vi "GDSLvIcon_GenerateObjectIcon.vi"(1 "HeaderColor":u32(colorbox)=786176, 3 "BackgroundColor":u32(colorbox)=16775072, 4 "Height":u32=22, 5 "error in (no error)":errorcluster, 6 "Type":enum16{"LvClass", "Library", "X-Control"}(ring), 7 "Width(30)":u32=30, 8 "ClassBodyIcon":string, 9 "_Thickness":u8=1 caption="Thickness (pixels)" min=1 max=3 step=1) -> (15 "BodyIconOut":u8[][](array[numeric])=[[2, 2, 2, 2, 2, 2, 2, 2, 2, 2, 2, 2, 2, 2, 2, 2, 2, 2, 2, 2, 2, 2, 2, 2, 2, 2, 2, 2, 2, 2], [2, 2, 2, 2, 2, 2, 2, 2, 2, 2, 2, 2, 2, 2, 185, 185, 2, 2, 2, 2, 2, 2, 2, 2, 2, 2, 2, 2, 2, 2], [2, 2, 2, 2, 2, 2, 2, 2, 2, 2, 2, 2, 185, 229, 227, 229, 229, 185, 2, 2, 2, 2, 2, 2, 2, 2, 2, 2, 2, 2], [2, 2, 2, 2, 2, 2, 2, 2, 2, 2, 185, 229, 227, 185, 185, 185, 185, 229, 229, 185, 2, 2, 2, 2, 2, 2, 2, 2, 2, 2], [2, 2, 2, 2, 2, 2, 2, 2, 185, 229, 227, 185, 185, 185, 185, 185, 185, 185, 185, 229, 229, 185, 2, 2, 2, 2, 2, 2, 2, 2], [2, 2, 2, 2, 2, 2, 2, 229, 227, 185, 185, 185, 185, 185, 185, 185, 185, 185, 185, 185, 185, 229, 229, 2, 2, 2, 2, 2, 2, 2], [2, 2, 2, 2, 2, 2, 2, 227, 227, 185, 185, 185, 185, 185, 185, 185, 185, 185, 185, 185, 185, 232, 229, 2, 2, 2, 2, 2, 2, 2], [2, 2, 2, 2, 2, 2, 2, 227, 229, 229, 227, 185, 185, 185, 185, 185, 185, 185, 185, 232, 232, 232, 227, 2, 2, 2, 2, 2, 2, 2], [2, 2, 2, 2, 2, 2, 2, 227, 229, 229, 229, 229, 227, 185, 185, 185, 185, 232, 232, 232, 232, 232, 227, 2, 2, 2, 2, 2, 2, 2], [2, 2, 2, 2, 2, 2, 2, 227, 229, 229, 229, 229, 229, 229, 227, 229, 232, 232, 232, 232, 232, 232, 227, 2, 2, 2, 2, 2, 2, 2], [2, 2, 2, 2, 2, 2, 2, 227, 229, 229, 229, 229, 229, 229, 229, 232, 232, 232, 232, 232, 232, 232, 227, 2, 2, 2, 2, 2, 2, 2], [2, 2, 2, 2, 2, 2, 2, 227, 229, 229, 229, 229, 229, 229, 229, 232, 232, 232, 232, 232, 232, 232, 227, 2, 2, 2, 2, 2, 2, 2], [2, 2, 2, 2, 2, 2, 2, 227, 229, 229, 229, 229, 229, 229, 229, 232, 232, 232, 232, 232, 232, 232, 227, 2, 2, 2, 2, 2, 2, 2], [2, 2, 2, 2, 2, 2, 2, 227, 229, 229, 229, 229, 229, 229, 229, 232, 232, 232, 232, 232, 232, 232, 227, 2, 2, 2, 2, 2, 2, 2], [2, 2, 2, 2, 2, 2, 2, 227, 229, 229, 229, 229, 229, 229, 229, 232, 232, 232, 232, 232, 232, 232, 227, 2, 2, 2, 2, 2, 2, 2], [2, 2, 2, 2, 2, 2, 2, 229, 229, 229, 229, 229, 229, 229, 229, 232, 232, 232, 232, 232, 232, 229, 229, 172, 172, 172, 2, 2, 2, 2], [2, 2, 2, 2, 2, 2, 2, 2, 227, 227, 229, 229, 229, 229, 229, 232, 232, 232, 232, 229, 229, 227, 172, 172, 172, 172, 172, 172, 2, 2], [2, 2, 2, 2, 2, 2, 2, 2, 2, 2, 227, 229, 229, 229, 229, 232, 232, 229, 229, 227, 172, 172, 172, 172, 172, 172, 2, 2, 2, 2], [2, 2, 2, 2, 2, 2, 2, 2, 2, 2, 2, 2, 227, 229, 229, 229, 229, 185, 172, 172, 172, 172, 172, 172, 172, 2, 2, 2, 2, 2], [2, 2, 2, 2, 2, 2, 2, 2, 2, 2, 2, 2, 2, 2, 227, 185, 172, 172, 172, 172, 172, 172, 172, 2, 2, 2, 2, 2, 2, 2], [2, 2, 2, 2, 2, 2, 2, 2, 2, 2, 2, 2, 2, 2, 2, 2, 2, 172, 172, 172, 172, 2, 2, 2, 2, 2, 2, 2, 2, 2], [2, 2, 2, 2, 2, 2, 2, 2, 2, 2, 2, 2, 2, 2, 2, 2, 2, 2, 2, 2, 2, 2, 2, 2, 2, 2, 2, 2, 2, 2]] format="%x", 19 "error out":errorcluster)   [LabVIEW 2020]
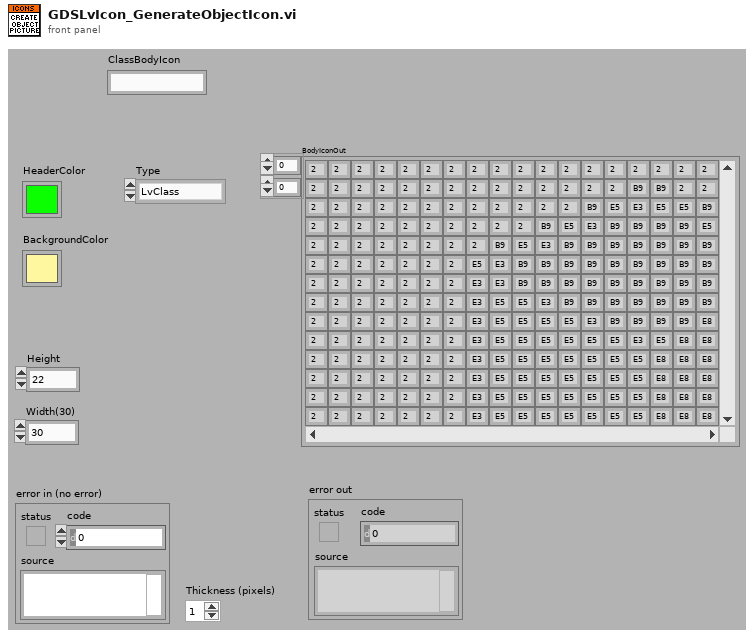
[diagram p1: front panel]
types:
  T1 = typedef "imagedata.ctl" = cluster{"image type":i32, "image depth":i32, "image":u8[], "mask":u8[], "colors":u32[], "Rectangle":cluster{"left":i16, "top":i16, "right":i16, "bottom":i16}}
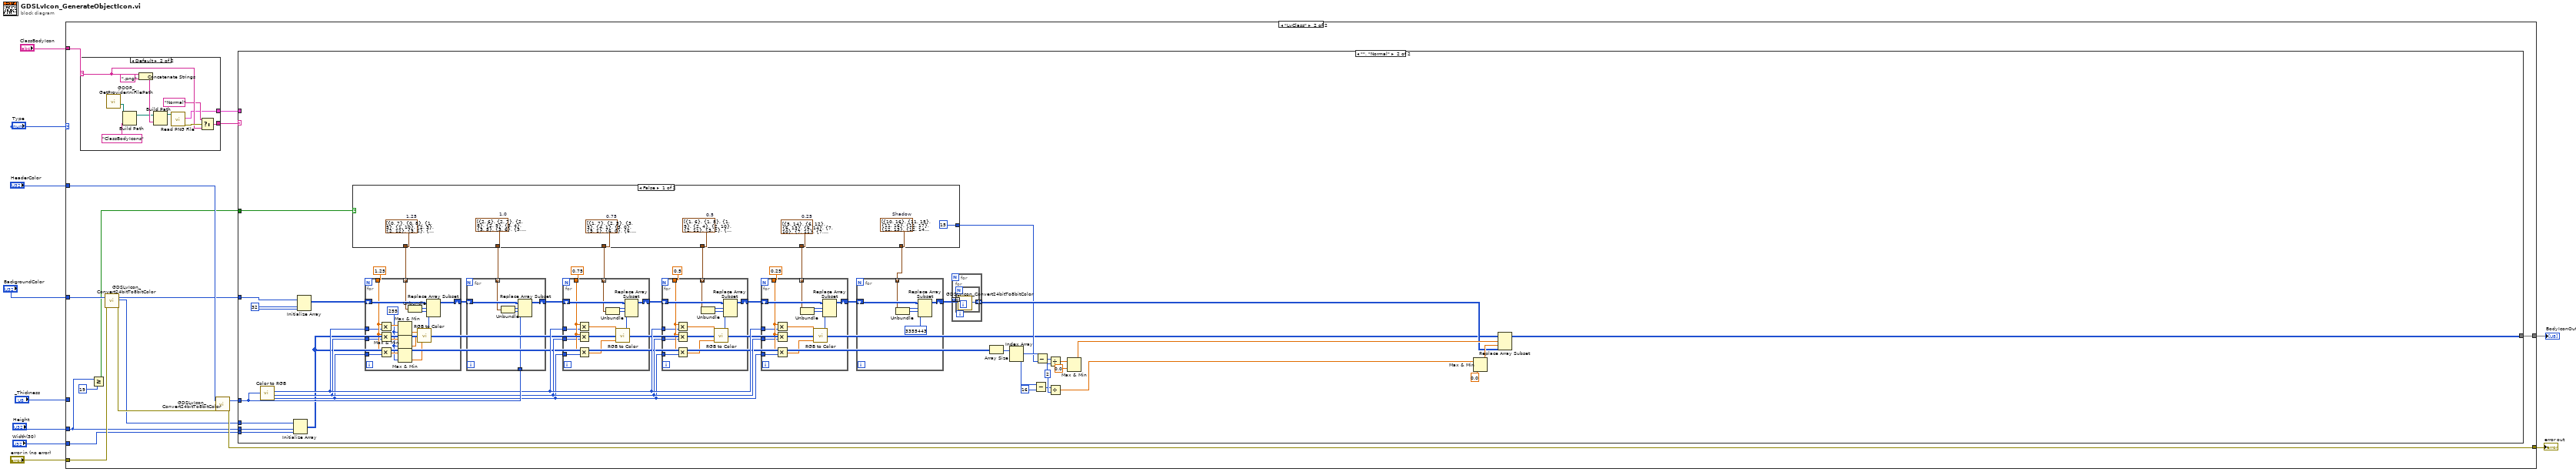
[diagram p0: block diagram]
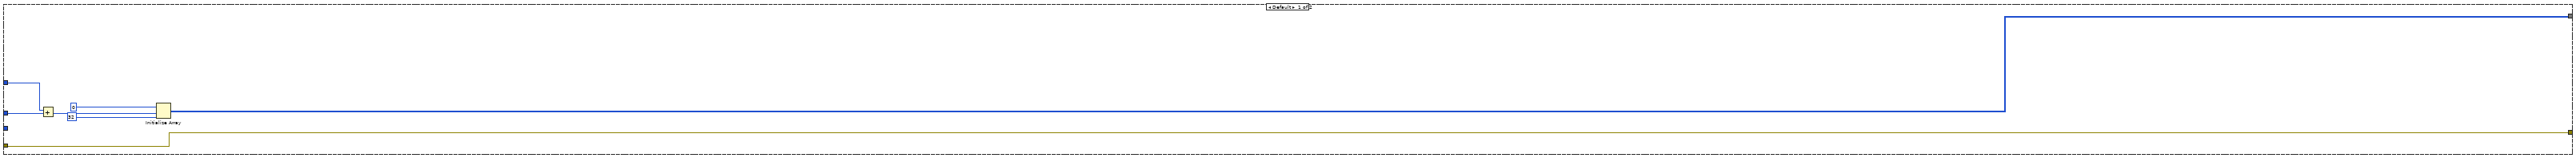
[diagram p2: hidden frame]
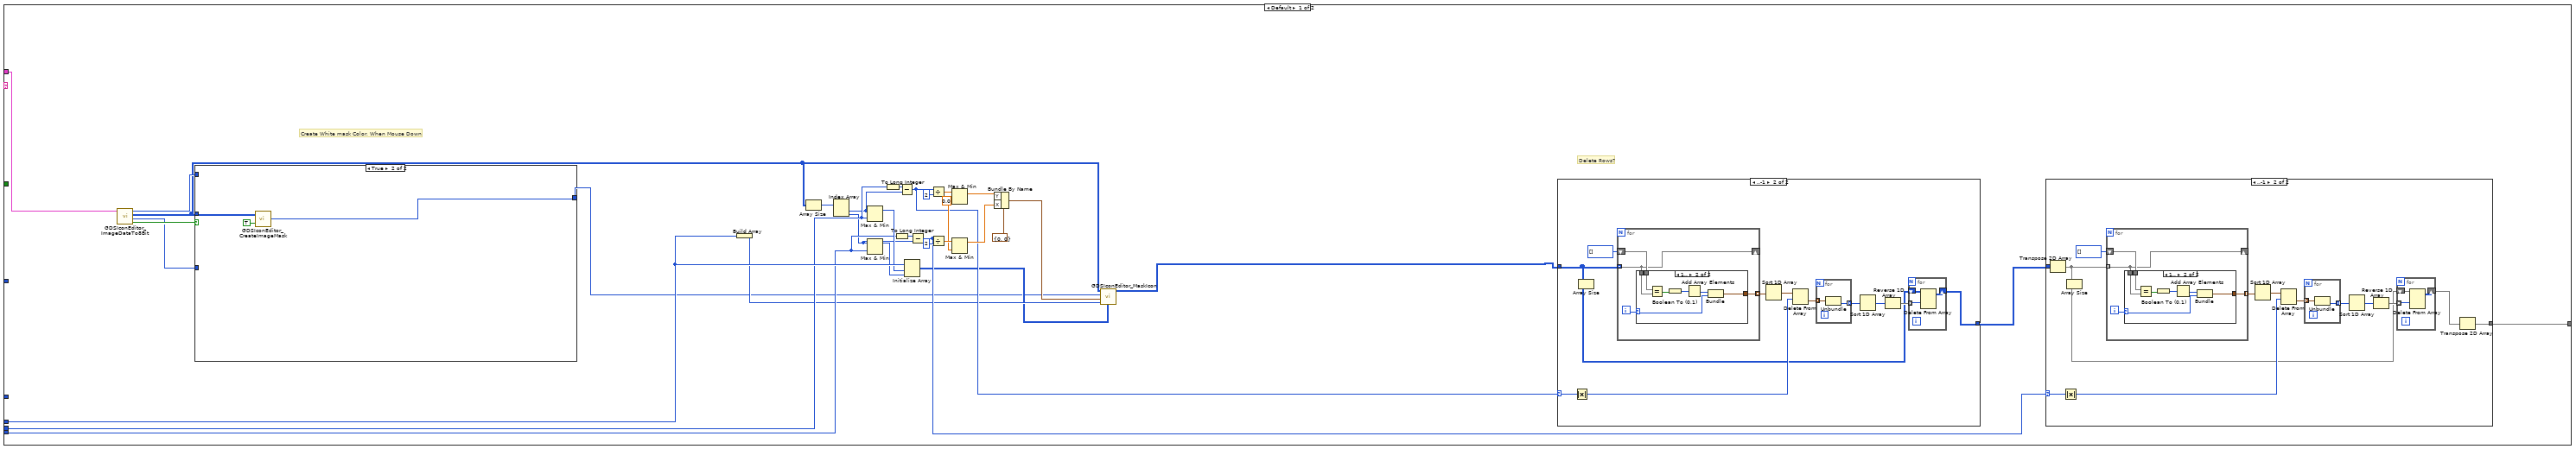
[diagram p4: hidden frame]
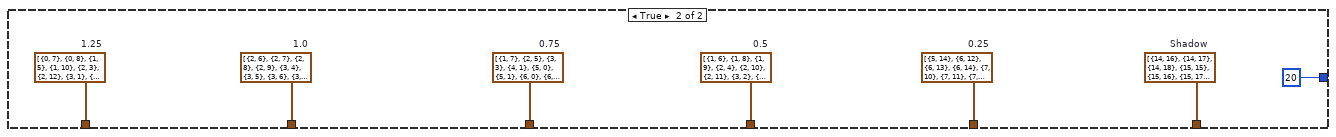
[diagram p10: hidden frame]
diagram:
  n1 = case shown="\"LvClass\"" "Type" {
    tunnel: "HeaderColor" -> [_ w33]
    tunnel: [w15 w31] -> w9
    tunnel: "BackgroundColor" -> [_ w30]
    tunnel: "error in (no error)" -> [w15 w29]
    tunnel: "Width(30)" -> [_ w18]
    tunnel: "Height" -> [w13 w19]
    tunnel: [w16 w22] -> w4
    tunnel: "_Thickness" -> [w12 _]
    tunnel: "ClassBodyIcon" -> [_ w24]
    frame Default {
      n2 = Add(x=w12, y=w13) -> (x+y=w11:u32)
      n3 = Initialize Array(u8 0 ("element"), w11, 32 ("dimension size")) -> (w16:u8[][])
    }
    frame "LvClass" {
      n4 = case shown="Default" w24 {
        selector: w24 -> [w34 w38]
        tunnel: [w34 w37] -> w23
        tunnel: [_ w35] -> w21
        frame "", "Normal" {
        }
        frame Default {
          n5 = call <resource>:"GOOP_GetProviderIniFilePath.vi"() -> ("ProviderMainFolder"=w42:path)  [unwired: 10 in, 1 out]
          n6 = Build Path(base path=w42, name or relative path="ClassBodyIcons") -> (appended path=w44:path)
          n7 = Concatenate Strings(w38, ".png" ("string")) -> (w45:string)
          n8 = Build Path(base path=w44, name or relative path=w45) -> (appended path=w40:path)
          n9 = call <vilib>:"Read PNG File.vi"("path to PNG file"=w40) -> ("error out"=w39:errorcluster, "image data"=w35:T1)  [unwired: 8 in, 1 out]
          n10 = Select(t="Normal", s=w39, f=w38) -> (s? t:f=w37:string)
        }
      }
      n11 = Greater Or Equal?(x=w19, y=19) -> (x >= y?=w26:bool)
      n12 = call <resource>:"GDSLvIcon_Convert24bitTo8bitColor.vi"("Color 24bit In"=w30, "error in (no error)"=w29) -> ("Adjusted 24bit Color Out"=w25:u32, "Color out(256)"=w20:u8, "error out"=w28:errorcluster)  [unwired: 14 in, 1 out]
      n13 = call <resource>:"GDSLvIcon_Convert24bitTo8bitColor.vi"("Color 24bit In"=w33, "error in (no error)"=w28) -> ("Adjusted 24bit Color Out"=w32:u32, "error out"=w31:errorcluster)  [unwired: 14 in, 2 out]
      n14 = case shown="\"\", \"Normal\"" w23 {
        tunnel: w32 -> [_ w180]
        tunnel: w26 -> [_ w162]
        tunnel: w25 -> [_ w161]
        tunnel: [w53 w144] -> w22
        tunnel: w21 -> [w75 _]
        tunnel: w20 -> [w73 w143]
        tunnel: w19 -> [w70 w142]
        tunnel: w18 -> [w62 w141]
        frame Default {
          w59 = 0.0 ("y")
          # "Delete Rows?"
          # "Create White mask Color, When Mouse Down"
          n15 = call <resource>:"GDSIconEditor_ImageDataTo8Bit.vi"("image data"=w75) -> ("NoMaskFound"=w77:bool, "ColorArray"=w52:u32[], "8-bit pixmap"=w49:u8[][], "mask"=w76:u8[])  [unwired: 7 in]
          n16 = case shown="True" w77 {
            tunnel: w49 -> [_ w139]
            tunnel: w76 -> [w136 _]
            tunnel: [w136 w137] -> w46
            tunnel: w52 -> [_ _]
            frame False {
            }
            frame True {
              n17 = call <resource>:"GDSIconEditor_CreateImageMask.vi"("Flood Fill"=TRUE, "8-bit pixmap"=w139) -> ("Array"=w137:u8[])
            }
          }
          n18 = Build Array(w73) -> (w50:u8[])
          n19 = Array Size(array=w49) -> (size(s)=w74:i32[])
          n20 = Index Array(array=w74) -> (element #1=w69:i32, element #2=w61:i32)  [unwired: 2 in]
          n21 = Max & Min(x=w69, y=w70) -> (max(x,y)=w72:u32)  [unwired: 1 out]
          n22 = Max & Min(x=w61, y=w62) -> (max(x,y)=w71:u32)  [unwired: 1 out]
          n23 = To Long Integer(number=w70) -> (32bit integer=w58:i32)
          n24 = To Long Integer(number=w62) -> (32bit integer=w57:i32)
          n25 = Subtract(x=w58, y=w69) -> (x-y=w56:i32)
          n26 = Initialize Array(w73, w72, w71) -> (w47:u8[][])
          n27 = Subtract(x=w57, y=w61) -> (x-y=w54:i32)
          n28 = Divide(x=w56, y=u32 2) -> (x/y=w67:dbl)
          n29 = Divide(x=w54, y=u32 2) -> (x/y=w64:dbl)
          n30 = Max & Min(x=w67, y=w59) -> (max(x,y)=w65:dbl)  [unwired: 1 out]
          n31 = Max & Min(x=w64, y=w59) -> (max(x,y)=w60:dbl)  [unwired: 1 out]
          n32 = Bundle By Name(cluster=cluster{"X":i32, "Y":i32} {"X"=0, "Y"=0} ("BgIconOffset"), "Y"=w65, "X"=w60) -> (w51:cluster{"X":i32, "Y":i32})
          n33 = call <resource>:"GDSIconEditor_MaskIcon.vi"("BgIcon"=w47, "ColorsOkayforiconToBeOnTopOf"=w50, "BgIconOffset"=w51, "BgIconMask"=w46, "IconIn"=w49) -> ("IconOut"=w48:u8[][])  [unwired: 6 in]
          n34 = case shown="..-1" w56 {
            selector: w56 -> [_ w119]
            tunnel: w48 -> [w108 w109]
            tunnel: [w108 w110] -> w55
            frame Default {
            }
            frame ..-1 {
              n35 = Absolute Value(x=w119) -> (abs(x)=w115:i32)
              n36 = Array Size(array=w109) -> ()  [unwired: 1 out]
              n37 = for {
                tunnel: w109 -> [w126] mode=indexing
                shift-right: [w126] -> _
                shift-left: u8[] [] -> [w127]
                tunnel: [w125] -> w117 mode=indexing
                i -> [w128]
                n38 = case shown="1.." w128 {
                  selector: w128 -> [_ w130]
                  tunnel: w127 -> [_ w135]
                  tunnel: w126 -> [_ w134]
                  tunnel: [_ w129] -> w125
                  frame 0, Default {
                  }
                  frame 1.. {
                    n39 = Equal?(x=w135, y=w134) -> (x = y?=w133:bool[])
                    n40 = Boolean To (0,1)(Boolean=w133) -> (0, 1=w132:i16[])
                    n41 = Add Array Elements(numeric array=w132) -> (sum=w131:i16)
                    n42 = Bundle("Color out(256)"=w131, w130) -> (w129:cluster{"Color out(256)":i16, i32})  [unwired: 1 in]
                  }
                }
              }
              n43 = Sort 1D Array(array=w117) -> (sorted array=w116:cluster{"Color out(256)":i16, i32}[])
              n44 = Delete From Array(array=w116, length=w115) -> (deleted portion=w114:cluster{"Color out(256)":i16, i32}[])  [unwired: 1 in, 1 out]
              n45 = for {
                tunnel: w114 -> [w124] mode=indexing
                tunnel: [w123] -> w113 mode=indexing
                n46 = Unbundle(w124) -> (w123:i32)  [unwired: 1 out]
              }
              n47 = Sort 1D Array(array=w113) -> (sorted array=w112:i32[])
              n48 = Reverse 1D Array(array=w112) -> (reversed array=w111:i32[])
              n49 = for {
                tunnel: w111 -> [w120] mode=indexing
                shift-right: [w121] -> w110
                shift-left: w109 -> [w122]
                n50 = Delete From Array(array=w122, index (row)=w120) -> (array with subset deleted=w121:u8[][])  [unwired: 2 in, 1 out]
              }
            }
          }
          n51 = case shown="..-1" w54 {
            selector: w54 -> [_ w91]
            tunnel: w55 -> [w78 w81]
            tunnel: [w78 w79] -> w53
            frame Default {
            }
            frame ..-1 {
              n52 = Transpose 2D Array(2D array=w81) -> (transposed array=w80:u8[][])
              n53 = Absolute Value(x=w91) -> (abs(x)=w87:i32)
              n54 = Array Size(array=w80) -> ()  [unwired: 1 out]
              n55 = for {
                tunnel: w80 -> [w98] mode=indexing
                shift-right: [w98] -> _
                shift-left: u8[] [] -> [w99]
                tunnel: [w97] -> w89 mode=indexing
                i -> [w100]
                n56 = case shown="1.." w100 {
                  selector: w100 -> [_ w102]
                  tunnel: w99 -> [_ w107]
                  tunnel: w98 -> [_ w106]
                  tunnel: [_ w101] -> w97
                  frame 0, Default {
                  }
                  frame 1.. {
                    n57 = Equal?(x=w107, y=w106) -> (x = y?=w105:bool[])
                    n58 = Boolean To (0,1)(Boolean=w105) -> (0, 1=w104:i16[])
                    n59 = Add Array Elements(numeric array=w104) -> (sum=w103:i16)
                    n60 = Bundle("Color out(256)"=w103, w102) -> (w101:cluster{"Color out(256)":i16, i32})  [unwired: 1 in]
                  }
                }
              }
              n61 = Sort 1D Array(array=w89) -> (sorted array=w88:cluster{"Color out(256)":i16, i32}[])
              n62 = Delete From Array(array=w88, length=w87) -> (deleted portion=w86:cluster{"Color out(256)":i16, i32}[])  [unwired: 1 in, 1 out]
              n63 = for {
                tunnel: w86 -> [w96] mode=indexing
                tunnel: [w95] -> w85 mode=indexing
                n64 = Unbundle(w96) -> (w95:i32)  [unwired: 1 out]
              }
              n65 = Sort 1D Array(array=w85) -> (sorted array=w84:i32[])
              n66 = Reverse 1D Array(array=w84) -> (reversed array=w83:i32[])
              n67 = for {
                tunnel: w83 -> [w92] mode=indexing
                shift-right: [w93] -> w82
                shift-left: w80 -> [w94]
                n68 = Delete From Array(array=w94, index (row)=w92) -> (array with subset deleted=w93:u8[][])  [unwired: 2 in, 1 out]
              }
              n69 = Transpose 2D Array(2D array=w82) -> (transposed array=w79:u8[][])
            }
          }
        }
        frame "", "Normal" {
          w151 = 2 ("y")
          w169 = 32 ("dimension size")
          n70 = call <vilib>:"Color to RGB.vi"("Color"=w180) -> ("R"=w172:u8, "G"=w171:u8, "B"=w170:u8)  [unwired: 1 out]
          n71 = Initialize Array(w143, w142, w141) -> (w140:u8[][])
          n72 = Initialize Array(w161, w169, w169) -> (w183:u32[][])
          n73 = case shown="False" w162 {
            tunnel: [w189 w201] -> w168
            tunnel: [w190 w200] -> w167
            tunnel: [w191 w199] -> w166
            tunnel: [w192 w198] -> w165
            tunnel: [w193 w197] -> w164
            tunnel: [w194 w196] -> w163
            tunnel: [15 ("y") 20 ("y")] -> w145
            frame False {
              w189 = cluster{"X":i32, "Y":i32}[] [{"X"=0, "Y"=7}, {"X"=0, "Y"=8}, {"X"=1, "Y"=5}, {"X"=1, "Y"=10}, {"X"=2, "Y"=3}, {"X"=2, "Y"=12}, {"X"=3, "Y"=1}, {"X"=3, "Y"=14}]  # 1.25
              w190 = cluster{"X":i32, "Y":i32}[] [{"X"=2, "Y"=6}, {"X"=2, "Y"=7}, {"X"=2, "Y"=8}, {"X"=2, "Y"=9}, {"X"=3, "Y"=4}, {"X"=3, "Y"=5}, {"X"=3, "Y"=6}, {"X"=3, "Y"=7}, {"X"=3, "Y"=8}, {"X"=3, "Y"=9}, {"X"=3, "Y"=10}, {"X"=3, "Y"=11}, {"X"=4, "Y"=2}, {"X"=4, "Y"=3}, {"X"=4, "Y"=4}, {"X"=4, "Y"=5}, {"X"=4, "Y"=6}, {"X"=4, "Y"=7}, {"X"=4, "Y"=8}, {"X"=4, "Y"=9}, {"X"=4, "Y"=10}, {"X"=4, "Y"=11}, {"X"=4, "Y"=12}, {"X"=4, "Y"=13}, {"X"=5, "Y"=2}, {"X"=5, "Y"=3}, {"X"=5, "Y"=4}, {"X"=5, "Y"=5}, {"X"=5, "Y"=6}, {"X"=5, "Y"=7}, {"X"=5, "Y"=8}, {"X"=5, "Y"=9}, {"X"=5, "Y"=10}, {"X"=5, "Y"=11}, {"X"=5, "Y"=12}, {"X"=5, "Y"=13}, {"X"=6, "Y"=4}, {"X"=6, "Y"=5}, {"X"=6, "Y"=6}, {"X"=6, "Y"=7}, {"X"=6, "Y"=8}, {"X"=6, "Y"=9}, {"X"=6, "Y"=10}, {"X"=6, "Y"=11}, {"X"=7, "Y"=6}, {"X"=7, "Y"=7}, {"X"=7, "Y"=8}, {"X"=7, "Y"=9}, {"X"=13, "Y"=10}, {"X"=14, "Y"=8}]  # 1.0
              w192 = cluster{"X":i32, "Y":i32}[] [{"X"=1, "Y"=6}, {"X"=1, "Y"=8}, {"X"=1, "Y"=9}, {"X"=2, "Y"=4}, {"X"=2, "Y"=10}, {"X"=2, "Y"=11}, {"X"=3, "Y"=2}, {"X"=3, "Y"=12}, {"X"=3, "Y"=13}, {"X"=4, "Y"=0}, {"X"=4, "Y"=14}, {"X"=4, "Y"=15}, {"X"=5, "Y"=15}, {"X"=6, "Y"=1}, {"X"=6, "Y"=2}, {"X"=7, "Y"=1}, {"X"=7, "Y"=2}, {"X"=7, "Y"=3}, {"X"=7, "Y"=4}, {"X"=8, "Y"=1}, {"X"=8, "Y"=2}, {"X"=8, "Y"=3}, {"X"=8, "Y"=4}, {"X"=8, "Y"=5}, {"X"=8, "Y"=6}, {"X"=8, "Y"=8}, {"X"=9, "Y"=1}, {"X"=9, "Y"=2}, {"X"=9, "Y"=3}, {"X"=9, "Y"=4}, {"X"=9, "Y"=5}, {"X"=9, "Y"=6}, {"X"=9, "Y"=7}, {"X"=10, "Y"=0}, {"X"=10, "Y"=1}, {"X"=10, "Y"=2}, {"X"=10, "Y"=3}, {"X"=10, "Y"=4}, {"X"=10, "Y"=5}, {"X"=10, "Y"=6}, {"X"=10, "Y"=7}, {"X"=10, "Y"=14}, {"X"=10, "Y"=15}, {"X"=11, "Y"=3}, {"X"=11, "Y"=4}, {"X"=11, "Y"=5}, {"X"=11, "Y"=6}, {"X"=11, "Y"=7}, {"X"=11, "Y"=12}, {"X"=11, "Y"=13}, {"X"=12, "Y"=4}, {"X"=12, "Y"=5}, {"X"=12, "Y"=6}, {"X"=12, "Y"=7}, {"X"=12, "Y"=10}, {"X"=12, "Y"=11}, {"X"=13, "Y"=6}, {"X"=13, "Y"=7}, {"X"=13, "Y"=8}, {"X"=13, "Y"=9}]  # 0.5
              w191 = cluster{"X":i32, "Y":i32}[] [{"X"=1, "Y"=7}, {"X"=2, "Y"=5}, {"X"=3, "Y"=3}, {"X"=4, "Y"=1}, {"X"=5, "Y"=0}, {"X"=5, "Y"=1}, {"X"=6, "Y"=0}, {"X"=6, "Y"=3}, {"X"=6, "Y"=15}, {"X"=7, "Y"=0}, {"X"=7, "Y"=5}, {"X"=7, "Y"=15}, {"X"=8, "Y"=0}, {"X"=8, "Y"=7}, {"X"=8, "Y"=15}, {"X"=9, "Y"=0}, {"X"=9, "Y"=15}, {"X"=11, "Y"=1}, {"X"=11, "Y"=2}, {"X"=11, "Y"=14}, {"X"=12, "Y"=3}, {"X"=12, "Y"=12}, {"X"=13, "Y"=5}, {"X"=14, "Y"=7}]  # 0.75
              w193 = cluster{"X":i32, "Y":i32}[] [{"X"=5, "Y"=14}, {"X"=6, "Y"=12}, {"X"=6, "Y"=13}, {"X"=6, "Y"=14}, {"X"=7, "Y"=10}, {"X"=7, "Y"=11}, {"X"=7, "Y"=12}, {"X"=7, "Y"=13}, {"X"=7, "Y"=14}, {"X"=8, "Y"=9}, {"X"=8, "Y"=10}, {"X"=8, "Y"=11}, {"X"=8, "Y"=12}, {"X"=8, "Y"=13}, {"X"=8, "Y"=14}, {"X"=9, "Y"=8}, {"X"=9, "Y"=9}, {"X"=9, "Y"=10}, {"X"=9, "Y"=11}, {"X"=9, "Y"=12}, {"X"=9, "Y"=13}, {"X"=9, "Y"=14}, {"X"=10, "Y"=8}, {"X"=10, "Y"=9}, {"X"=10, "Y"=10}, {"X"=10, "Y"=11}, {"X"=10, "Y"=12}, {"X"=10, "Y"=13}, {"X"=11, "Y"=8}, {"X"=11, "Y"=9}, {"X"=11, "Y"=10}, {"X"=11, "Y"=11}, {"X"=12, "Y"=8}, {"X"=12, "Y"=9}]  # 0.25
              w194 = cluster{"X":i32, "Y":i32}[] [{"X"=10, "Y"=16}, {"X"=11, "Y"=15}, {"X"=11, "Y"=16}, {"X"=11, "Y"=17}, {"X"=12, "Y"=13}, {"X"=12, "Y"=14}, {"X"=12, "Y"=15}, {"X"=12, "Y"=16}, {"X"=12, "Y"=17}, {"X"=13, "Y"=11}, {"X"=13, "Y"=12}, {"X"=13, "Y"=13}, {"X"=13, "Y"=14}, {"X"=13, "Y"=15}, {"X"=13, "Y"=16}, {"X"=14, "Y"=9}, {"X"=14, "Y"=10}, {"X"=14, "Y"=11}, {"X"=14, "Y"=12}, {"X"=14, "Y"=13}, {"X"=14, "Y"=14}, {"X"=14, "Y"=15}, {"X"=15, "Y"=10}, {"X"=15, "Y"=11}, {"X"=15, "Y"=12}, {"X"=15, "Y"=13}]  # Shadow
            }
            frame True {
              w196 = cluster{"X":i32, "Y":i32}[] [{"X"=14, "Y"=16}, {"X"=14, "Y"=17}, {"X"=14, "Y"=18}, {"X"=15, "Y"=15}, {"X"=15, "Y"=16}, {"X"=15, "Y"=17}, {"X"=15, "Y"=18}, {"X"=15, "Y"=19}, {"X"=15, "Y"=20}, {"X"=16, "Y"=13}, {"X"=16, "Y"=14}, {"X"=16, "Y"=15}, {"X"=16, "Y"=16}, {"X"=16, "Y"=17}, {"X"=16, "Y"=18}, {"X"=17, "Y"=11}, {"X"=17, "Y"=12}, {"X"=17, "Y"=13}, {"X"=17, "Y"=14}, {"X"=17, "Y"=15}, {"X"=17, "Y"=16}, {"X"=17, "Y"=17}, {"X"=18, "Y"=9}, {"X"=18, "Y"=10}, {"X"=18, "Y"=11}, {"X"=18, "Y"=12}, {"X"=18, "Y"=13}, {"X"=18, "Y"=14}, {"X"=18, "Y"=15}, {"X"=19, "Y"=10}, {"X"=19, "Y"=11}, {"X"=19, "Y"=12}, {"X"=19, "Y"=13}]  # Shadow
              w197 = cluster{"X":i32, "Y":i32}[] [{"X"=5, "Y"=14}, {"X"=6, "Y"=12}, {"X"=6, "Y"=13}, {"X"=6, "Y"=14}, {"X"=7, "Y"=10}, {"X"=7, "Y"=11}, {"X"=7, "Y"=12}, {"X"=7, "Y"=13}, {"X"=7, "Y"=14}, {"X"=8, "Y"=9}, {"X"=8, "Y"=10}, {"X"=8, "Y"=11}, {"X"=8, "Y"=12}, {"X"=8, "Y"=13}, {"X"=8, "Y"=14}, {"X"=9, "Y"=8}, {"X"=9, "Y"=9}, {"X"=9, "Y"=10}, {"X"=9, "Y"=11}, {"X"=9, "Y"=12}, {"X"=9, "Y"=13}, {"X"=9, "Y"=14}, {"X"=10, "Y"=8}, {"X"=10, "Y"=9}, {"X"=10, "Y"=10}, {"X"=10, "Y"=11}, {"X"=10, "Y"=12}, {"X"=10, "Y"=13}, {"X"=10, "Y"=14}, {"X"=11, "Y"=8}, {"X"=11, "Y"=9}, {"X"=11, "Y"=10}, {"X"=11, "Y"=11}, {"X"=11, "Y"=12}, {"X"=11, "Y"=13}, {"X"=11, "Y"=14}, {"X"=12, "Y"=8}, {"X"=12, "Y"=9}, {"X"=12, "Y"=10}, {"X"=12, "Y"=11}, {"X"=12, "Y"=12}, {"X"=12, "Y"=13}, {"X"=12, "Y"=14}, {"X"=13, "Y"=8}, {"X"=13, "Y"=9}, {"X"=13, "Y"=10}, {"X"=13, "Y"=11}, {"X"=13, "Y"=12}, {"X"=13, "Y"=13}, {"X"=13, "Y"=14}, {"X"=14, "Y"=8}, {"X"=14, "Y"=9}, {"X"=14, "Y"=10}, {"X"=14, "Y"=11}, {"X"=14, "Y"=12}, {"X"=14, "Y"=13}, {"X"=15, "Y"=8}, {"X"=15, "Y"=9}, {"X"=15, "Y"=10}, {"X"=15, "Y"=11}, {"X"=16, "Y"=8}, {"X"=16, "Y"=9}]  # 0.25
              w199 = cluster{"X":i32, "Y":i32}[] [{"X"=1, "Y"=7}, {"X"=2, "Y"=5}, {"X"=3, "Y"=3}, {"X"=4, "Y"=1}, {"X"=5, "Y"=0}, {"X"=5, "Y"=1}, {"X"=6, "Y"=0}, {"X"=6, "Y"=3}, {"X"=6, "Y"=15}, {"X"=7, "Y"=0}, {"X"=7, "Y"=5}, {"X"=7, "Y"=15}, {"X"=8, "Y"=0}, {"X"=8, "Y"=7}, {"X"=8, "Y"=15}, {"X"=9, "Y"=0}, {"X"=9, "Y"=15}, {"X"=10, "Y"=0}, {"X"=10, "Y"=15}, {"X"=11, "Y"=0}, {"X"=11, "Y"=15}, {"X"=12, "Y"=0}, {"X"=12, "Y"=15}, {"X"=13, "Y"=0}, {"X"=13, "Y"=15}, {"X"=15, "Y"=1}, {"X"=15, "Y"=2}, {"X"=15, "Y"=14}, {"X"=16, "Y"=3}, {"X"=16, "Y"=12}, {"X"=17, "Y"=5}, {"X"=18, "Y"=7}]  # 0.75
              w198 = cluster{"X":i32, "Y":i32}[] [{"X"=1, "Y"=6}, {"X"=1, "Y"=8}, {"X"=1, "Y"=9}, {"X"=2, "Y"=4}, {"X"=2, "Y"=10}, {"X"=2, "Y"=11}, {"X"=3, "Y"=2}, {"X"=3, "Y"=12}, {"X"=3, "Y"=13}, {"X"=4, "Y"=0}, {"X"=4, "Y"=14}, {"X"=4, "Y"=15}, {"X"=5, "Y"=15}, {"X"=6, "Y"=1}, {"X"=6, "Y"=2}, {"X"=7, "Y"=1}, {"X"=7, "Y"=2}, {"X"=7, "Y"=3}, {"X"=7, "Y"=4}, {"X"=8, "Y"=1}, {"X"=8, "Y"=2}, {"X"=8, "Y"=3}, {"X"=8, "Y"=4}, {"X"=8, "Y"=5}, {"X"=8, "Y"=6}, {"X"=8, "Y"=8}, {"X"=9, "Y"=1}, {"X"=9, "Y"=2}, {"X"=9, "Y"=3}, {"X"=9, "Y"=4}, {"X"=9, "Y"=5}, {"X"=9, "Y"=6}, {"X"=9, "Y"=7}, {"X"=10, "Y"=1}, {"X"=10, "Y"=2}, {"X"=10, "Y"=3}, {"X"=10, "Y"=4}, {"X"=10, "Y"=5}, {"X"=10, "Y"=6}, {"X"=10, "Y"=7}, {"X"=11, "Y"=1}, {"X"=11, "Y"=2}, {"X"=11, "Y"=3}, {"X"=11, "Y"=4}, {"X"=11, "Y"=5}, {"X"=11, "Y"=6}, {"X"=11, "Y"=7}, {"X"=12, "Y"=1}, {"X"=12, "Y"=2}, {"X"=12, "Y"=3}, {"X"=12, "Y"=4}, {"X"=12, "Y"=5}, {"X"=12, "Y"=6}, {"X"=12, "Y"=7}, {"X"=13, "Y"=1}, {"X"=13, "Y"=2}, {"X"=13, "Y"=3}, {"X"=13, "Y"=4}, {"X"=13, "Y"=5}, {"X"=13, "Y"=6}, {"X"=13, "Y"=7}, {"X"=14, "Y"=0}, {"X"=14, "Y"=1}, {"X"=14, "Y"=2}, {"X"=14, "Y"=3}, {"X"=14, "Y"=4}, {"X"=14, "Y"=5}, {"X"=14, "Y"=6}, {"X"=14, "Y"=7}, {"X"=14, "Y"=14}, {"X"=14, "Y"=15}, {"X"=15, "Y"=3}, {"X"=15, "Y"=4}, {"X"=15, "Y"=5}, {"X"=15, "Y"=6}, {"X"=15, "Y"=7}, {"X"=15, "Y"=12}, {"X"=15, "Y"=13}, {"X"=16, "Y"=4}, {"X"=16, "Y"=5}, {"X"=16, "Y"=6}, {"X"=16, "Y"=7}, {"X"=16, "Y"=10}, {"X"=16, "Y"=11}, {"X"=17, "Y"=6}, {"X"=17, "Y"=7}, {"X"=17, "Y"=8}, {"X"=17, "Y"=9}]  # 0.5
              w200 = cluster{"X":i32, "Y":i32}[] [{"X"=2, "Y"=6}, {"X"=2, "Y"=7}, {"X"=2, "Y"=8}, {"X"=2, "Y"=9}, {"X"=3, "Y"=4}, {"X"=3, "Y"=5}, {"X"=3, "Y"=6}, {"X"=3, "Y"=7}, {"X"=3, "Y"=8}, {"X"=3, "Y"=9}, {"X"=3, "Y"=10}, {"X"=3, "Y"=11}, {"X"=4, "Y"=2}, {"X"=4, "Y"=3}, {"X"=4, "Y"=4}, {"X"=4, "Y"=5}, {"X"=4, "Y"=6}, {"X"=4, "Y"=7}, {"X"=4, "Y"=8}, {"X"=4, "Y"=9}, {"X"=4, "Y"=10}, {"X"=4, "Y"=11}, {"X"=4, "Y"=12}, {"X"=4, "Y"=13}, {"X"=5, "Y"=2}, {"X"=5, "Y"=3}, {"X"=5, "Y"=4}, {"X"=5, "Y"=5}, {"X"=5, "Y"=6}, {"X"=5, "Y"=7}, {"X"=5, "Y"=8}, {"X"=5, "Y"=9}, {"X"=5, "Y"=10}, {"X"=5, "Y"=11}, {"X"=5, "Y"=12}, {"X"=5, "Y"=13}, {"X"=6, "Y"=4}, {"X"=6, "Y"=5}, {"X"=6, "Y"=6}, {"X"=6, "Y"=7}, {"X"=6, "Y"=8}, {"X"=6, "Y"=9}, {"X"=6, "Y"=10}, {"X"=6, "Y"=11}, {"X"=7, "Y"=6}, {"X"=7, "Y"=7}, {"X"=7, "Y"=8}, {"X"=7, "Y"=9}, {"X"=17, "Y"=10}, {"X"=18, "Y"=8}]  # 1.0
              w201 = cluster{"X":i32, "Y":i32}[] [{"X"=0, "Y"=7}, {"X"=0, "Y"=8}, {"X"=1, "Y"=5}, {"X"=1, "Y"=10}, {"X"=2, "Y"=3}, {"X"=2, "Y"=12}, {"X"=3, "Y"=1}, {"X"=3, "Y"=14}]  # 1.25
            }
          }
          n74 = for {
            shift-right: [w268] -> w181
            shift-left: w183 -> [w269]
            tunnel: w168 -> [w254] mode=indexing
            tunnel: 1.25 ("upper limit") -> [w260]
            tunnel: w172 -> [w259]
            tunnel: w171 -> [w258]
            tunnel: w170 -> [w257]
            w261 = 255 ("upper limit")
            n75 = Multiply(x=w260, y=w259) -> (x*y=w267:dbl)
            n76 = Multiply(x=w260, y=w258) -> (x*y=w263:dbl)
            n77 = Multiply(x=w260, y=w257) -> (x*y=w262:dbl)
            n78 = Max & Min(x=w267, y=w261) -> (min(x,y)=w266:dbl)  [unwired: 1 out]
            n79 = Max & Min(x=w263, y=w261) -> (min(x,y)=w265:dbl)  [unwired: 1 out]
            n80 = Max & Min(x=w262, y=w261) -> (min(x,y)=w264:dbl)  [unwired: 1 out]
            n81 = Unbundle(w254) -> ("X"=w255:i32, "Y"=w253:i32)
            n82 = call <vilib>:"RGB to Color.vi"("B"=w264, "G"=w265, "R"=w266) -> ("Color"=w256:u32)
            n83 = Replace Array Subset(array=w269, new element=w256, index (row)=w255, index (col)=w253) -> (w268:u32[][])
          }
          n84 = for {
            shift-right: [w251] -> w178
            shift-left: w181 -> [w252]
            tunnel: w167 -> [w250] mode=indexing
            tunnel: w180 -> [w249]
            n85 = Unbundle(w250) -> ("X"=w248:i32, "Y"=w247:i32)
            n86 = Replace Array Subset(array=w252, new element=w249, index (row)=w248, index (col)=w247) -> (w251:u32[][])
          }
          n87 = for {
            shift-right: [w245] -> w176
            shift-left: w178 -> [w246]
            tunnel: w166 -> [w244] mode=indexing
            tunnel: 0.75 ("upper limit") -> [w243]
            tunnel: w172 -> [w242]
            tunnel: w171 -> [w241]
            tunnel: w170 -> [w240]
            n88 = Multiply(x=w243, y=w242) -> (x*y=w238:dbl)
            n89 = Multiply(x=w243, y=w241) -> (x*y=w237:dbl)
            n90 = Multiply(x=w243, y=w240) -> (x*y=w236:dbl)
            n91 = Unbundle(w244) -> ("X"=w235:i32, "Y"=w234:i32)
            n92 = call <vilib>:"RGB to Color.vi"("B"=w236, "G"=w237, "R"=w238) -> ("Color"=w239:u32)
            n93 = Replace Array Subset(array=w246, new element=w239, index (row)=w235, index (col)=w234) -> (w245:u32[][])
          }
          n94 = for {
            shift-right: [w232] -> w174
            shift-left: w176 -> [w233]
            tunnel: w165 -> [w231] mode=indexing
            tunnel: 0.5 ("upper limit") -> [w230]
            tunnel: w172 -> [w229]
            tunnel: w171 -> [w228]
            tunnel: w170 -> [w227]
            n95 = Multiply(x=w230, y=w229) -> (x*y=w225:dbl)
            n96 = Multiply(x=w230, y=w228) -> (x*y=w224:dbl)
            n97 = Multiply(x=w230, y=w227) -> (x*y=w223:dbl)
            n98 = Unbundle(w231) -> ("X"=w222:i32, "Y"=w221:i32)
            n99 = call <vilib>:"RGB to Color.vi"("B"=w223, "G"=w224, "R"=w225) -> ("Color"=w226:u32)
            n100 = Replace Array Subset(array=w233, new element=w226, index (row)=w222, index (col)=w221) -> (w232:u32[][])
          }
          n101 = for {
            shift-right: [w219] -> w173
            shift-left: w174 -> [w220]
            tunnel: w164 -> [w218] mode=indexing
            tunnel: 0.25 ("upper limit") -> [w217]
            tunnel: w172 -> [w216]
            tunnel: w171 -> [w215]
            tunnel: w170 -> [w214]
            n102 = Multiply(x=w217, y=w216) -> (x*y=w212:dbl)
            n103 = Multiply(x=w217, y=w215) -> (x*y=w211:dbl)
            n104 = Multiply(x=w217, y=w214) -> (x*y=w210:dbl)
            n105 = Unbundle(w218) -> ("X"=w209:i32, "Y"=w208:i32)
            n106 = call <vilib>:"RGB to Color.vi"("B"=w210, "G"=w211, "R"=w212) -> ("Color"=w213:u32)
            n107 = Replace Array Subset(array=w220, new element=w213, index (row)=w209, index (col)=w208) -> (w219:u32[][])
          }
          n108 = for {
            shift-right: [w206] -> w160
            shift-left: w173 -> [w207]
            tunnel: w163 -> [w205] mode=indexing
            n109 = Unbundle(w205) -> ("X"=w203:i32, "Y"=w202:i32)
            n110 = Replace Array Subset(array=w207, new element=u32 3355443 ("new element/subarray"), index (row)=w203, index (col)=w202) -> (w206:u32[][])
          }
          n111 = for {
            tunnel: w160 -> [w185] mode=indexing
            tunnel: [w184] -> w146 mode=indexing
            n112 = for {
              tunnel: w185 -> [w187] mode=indexing
              tunnel: [w186] -> w184 mode=indexing
              n113 = call <resource>:"GDSLvIcon_Convert24bitTo8bitColor.vi"("Color 24bit In"=w187) -> ("Color out(256)"=w186:u8)  [unwired: 15 in, 3 out]
            }
          }
          n114 = Array Size(array=w140) -> (size(s)=w147:i32[])
          n115 = Index Array(array=w147) -> (element #1=w148:i32, element #2=w152:i32)  [unwired: 2 in]
          n116 = Subtract(x=w152, y=16) -> (x-y=w150:i32)
          n117 = Subtract(x=w148, y=w145) -> (x-y=w149:i32)
          n118 = Divide(x=w149, y=w151) -> (x/y=w155:dbl)
          n119 = Divide(x=w150, y=w151) -> (x/y=w158:dbl)
          n120 = Max & Min(x=w155, y=0.0) -> (max(x,y)=w156:dbl)  [unwired: 1 out]
          n121 = Max & Min(x=w158, y=0.0) -> (max(x,y)=w159:dbl)  [unwired: 1 out]
          n122 = Replace Array Subset(array=w140, new element=w146, index (row)=w156, index (col)=w159) -> (w144:u8[][])
        }
      }
    }
  }
  "error out" <- w9
  "BodyIconOut" <- w4
